vi "FugacityGraphWithTables.vi"(9 "Fugacity table":dbl[](array[numeric])=[0.0, 0.0], 10 "Temperature table":dbl[](array[numeric])=[0.0, 0.0]) -> (2 "XY Graph":cluster{ext[], ext[]}[](graph)=[{[17.44743958824043, 17.44743958824043], [-15.0, -45.0]}, {[14.85552997103172, 14.85552997103172], [-15.0, -45.0]}, {[12.93410075664489, 12.93410075664489], [-15.0, -45.0]}, {[11.45278589016778, 11.45278589016778], [-15.0, -45.0]}, {[10.2759081333812900003, 10.2759081333812900003], [-15.0, -45.0]}, {[9.318361831989936, 9.318361831989936], [-15.0, -45.0]}, {[9.0, 11.83374083129584, 18.0], [-17.9235, -25.63552567237164, -43.677999999999999999]}, {[0.0, 0.0], [0.0, 0.0]}])   [LabVIEW 2009]
panel:
  # "800"
  # "700"
  # "600"
  # "500"
  # "400"
  # "300"
  # "Temperature (*C)"
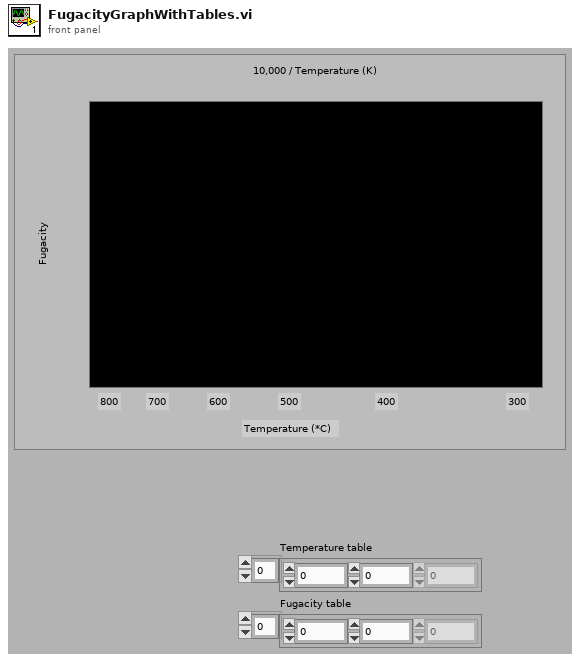
[diagram p1: front panel]
types:
  T1 = cluster{"Temperature table":dbl[], "Fugacity table":dbl[]}
  T2 = cluster{"Temperature table":dbl[], "Fugacity table":dbl[]}[]
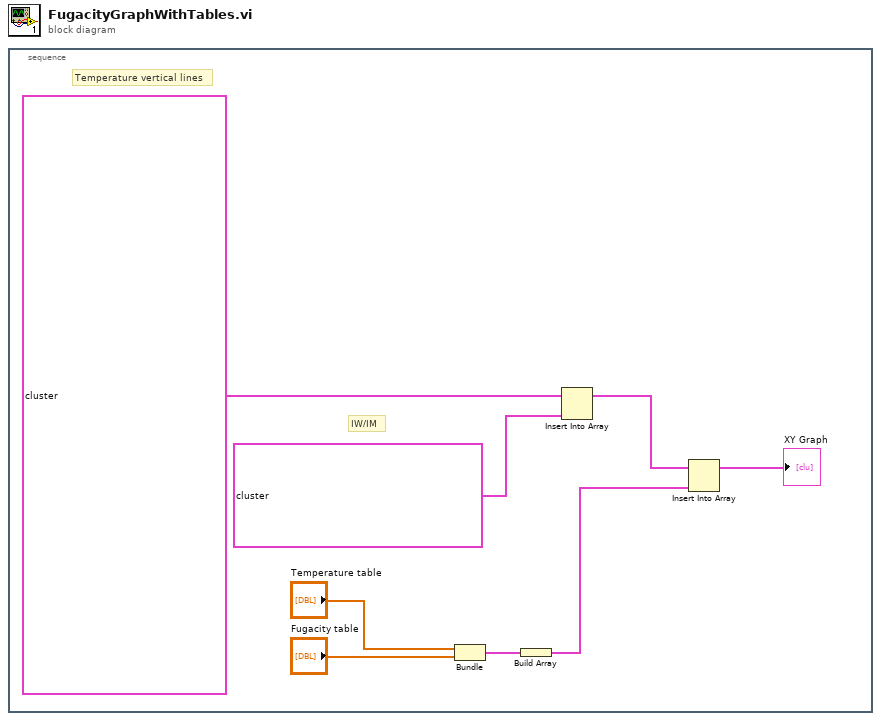
[diagram p0: block diagram]
diagram:
  n1 = stacked-sequence {
    frame #0 {
      # "IW/IM"
      # "Temperature vertical lines"
      n2 = Bundle("Temperature table"="Temperature table", "Fugacity table"="Fugacity table") -> (w3:T1)  [unwired: 1 in]
      n3 = Build Array(w3) -> (w4:T2)
      n4 = Insert Into Array(array=cluster{ext[], ext[]}[] [{[17.44743958824043, 17.44743958824043], [-15.0, -45.0]}, {[14.85552997103172, 14.85552997103172], [-15.0, -45.0]}, {[12.93410075664489, 12.93410075664489], [-15.0, -45.0]}, {[11.45278589016778, 11.45278589016778], [-15.0, -45.0]}, {[10.2759081333812900003, 10.2759081333812900003], [-15.0, -45.0]}, {[9.318361831989936, 9.318361831989936], [-15.0, -45.0]}], new element=cluster{ext[], ext[]}[] [{[9.0, 11.83374083129584, 18.0], [-17.9235, -25.63552567237164, -43.677999999999999999]}]) -> (w6:cluster{ext[], ext[]}[])  [unwired: 1 in]
      n5 = Insert Into Array(array=w6, new element=w4) -> (→"XY Graph":cluster{ext[], ext[]}[])  [unwired: 1 in]
    }
  }
